vi "Sandbox GUI.vi"() -> ()   [LabVIEW 2019]
uses:
  GUI_class/GUI.lvclass
  GUI Sensor Lib/GUI Sensor Lib.lvclass
  D:/LabASF/LabASF/src/GUI_class/GUI.lvclass
panel:
  out "dt":u32
  out "error out":errorcluster
  in  "remove":bool
  in  "insert":bool
  in  "close":bool
  in  "open":bool
  in  "stop":bool
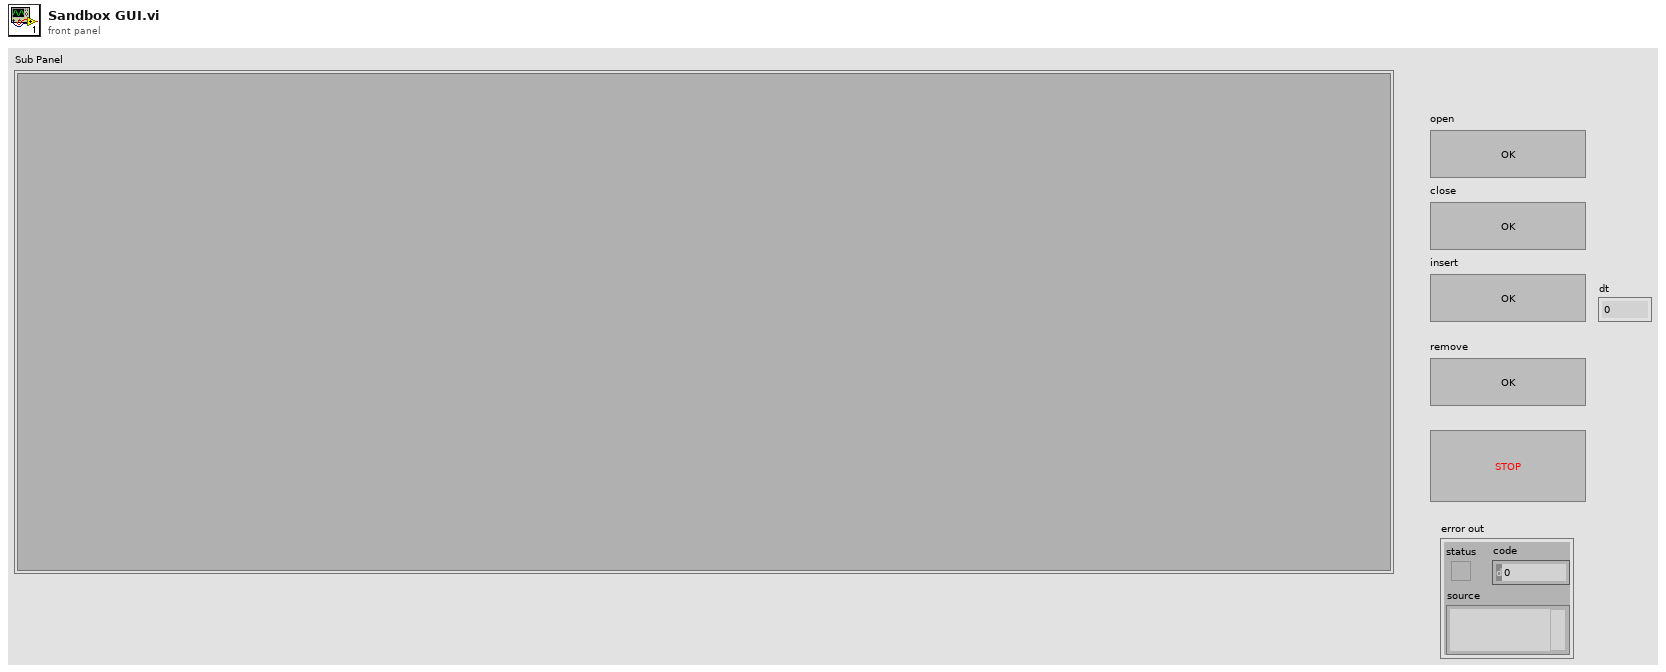
[diagram p1: front panel]
types:
  T1 = typedef "GUI Paths.ctl" = cluster{"Dir Data":path, "Dir Setting":path, "SensorLib":path, "Dir Scripts":path}
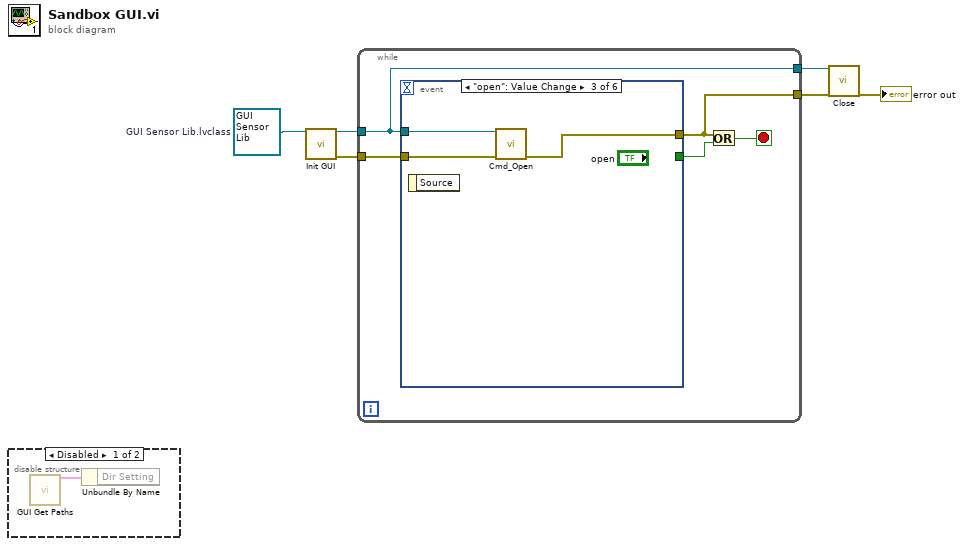
[diagram p0: block diagram]
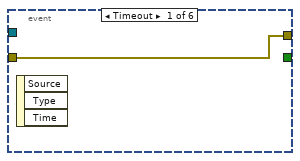
[diagram p3: hidden frame]
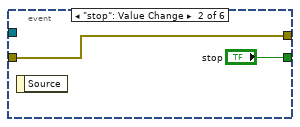
[diagram p4: hidden frame]
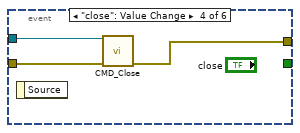
[diagram p5: hidden frame]
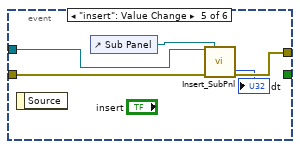
[diagram p6: hidden frame]
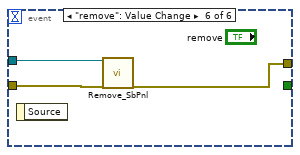
[diagram p7: hidden frame]
diagram:
  w1 = refnum<class "GUI Sensor Lib.lvclass"> refnum  # GUI Sensor Lib.lvclass
  n1 = disable-structure shown="Disabled" {
    frame Disabled {
      n2 = call "GUI Get Paths.vi"() -> ("Paths"=w7:T1)  [unwired: 14 in, 1 out]
      n3 = Unbundle By Name(w7) -> ()  [unwired: 1 out]
    }
    frame Enabled {
    }
  }
  n4 = call-dynamic "Init GUI.vi"("GUI in"=w1) -> ("GUI"=w6:refnum<class "GUI Sensor Lib.lvclass">, "error out"=w5:errorcluster)  [unwired: 12 in, 1 out]
  n5 = while {
    tunnel: w6 -> [w9]
    tunnel: w5 -> [w11]
    tunnel: [w9] -> w4
    tunnel: [w8] -> w3
    stop <- w10 stop-if-true
    n6 = event shown="[2] \"open\": Value Change" {
      selector: _ -> [_ _ _ _ _ _]
      dyn-events: _ -> [_ _ _ _ _ _]
      timeout: _ -> [_ _ _ _ _ _]
      tunnel: [_ "stop" _ _ _ _] -> w12
      tunnel: w9 -> [_ _ w17 w21 w26 w29]
      tunnel: w11 -> [w13 w14 w18 w20 w25 w28]
      tunnel: [w13 w14 w16 w19 w23 w27] -> w8
      event Timeout {
        n7 = event-data() -> ()  [unwired: 1 in, 3 out]
      }
      event "stop": Value Change {
        n8 = event-data() -> ()  [unwired: 1 in, 1 out]
      }
      event "open": Value Change {
        n9 = event-data() -> ()  [unwired: 1 in, 1 out]
        n10 = call "Cmd_Open.vi"("reference in"=w17, "error in (no error)"=w18) -> ("error out"=w16:errorcluster)  [unwired: 12 in, 1 out]
      }
      event "close": Value Change {
        n11 = event-data() -> ()  [unwired: 1 in, 1 out]
        n12 = call "CMD_Close.vi"("reference in"=w21, "error in (no error)"=w20) -> ("error out"=w19:errorcluster)  [unwired: 12 in, 1 out]
      }
      event "insert": Value Change {
        n13 = event-data() -> ()  [unwired: 1 in, 1 out]
        n14 = control-ref of="Sub Panel"() -> (w24:refnum<vi>)
        n15 = call "Insert_SubPnl.vi"("reference in"=w26, "SubPnl"=w24, "error in (no error)"=w25) -> ("dt"=→"dt":u32, "error out"=w23:errorcluster)  [unwired: 10 in, 1 out]
      }
      event "remove": Value Change {
        n16 = event-data() -> ()  [unwired: 1 in, 1 out]
        n17 = call "Remove_SbPnl.vi"("reference in"=w29, "error in (no error)"=w28) -> ("error out"=w27:errorcluster)  [unwired: 16 in, 1 out]
      }
    }
    n18 = Or(x=w8, y=w12) -> (x .or. y?=w10:bool)
  }
  n19 = call "Close.vi"("reference in"=w4, "error in (no error)"=w3) -> ("error out"=→"error out":errorcluster)  [unwired: 15 in, 2 out]
